vi "fpga_Sine Interpolation.vi"(6 "ready for output":bool, 8 "input valid":bool, 10 "Fnom":T1 items=["Fnom=50Hz", "Fnom=60Hz"], 11 "tach input":fxp<+/-,24,3> format="%.26g") -> (0 "output valid":bool, 1 "resampling valid":bool, 2 "crossing":fxp<+,32,16> format="%.21g", 3 "frequency":fxp<+,32,8> format="%.27g", 4 "ready for input":bool)   [LabVIEW 2011, in "NI_EP_Resample_FPGA.lvlib"]
uses:
  <vilib>/addons/Electrical Power/PQ/Resampling/NI_EP_Resample_FPGA.lvlib
  <vilib>/addons/Electrical Power/PQ/Resampling/FPGA/subVIs/fpga_Typedef Fnom.ctl
  <vilib>/rvi/FXPMathLib/basic elements/FxpIntAccumulator/subVIs/nifxpmath_IntAccumulator_SimConfig.ctl
  <vilib>/rvi/FXPMathLib/FxpSub/subVIs/nifxpmath_Sub_SimConfig.ctl
  <vilib>/fxp/LVFixedPointQuantizationPolicyTypeDef.ctl
  <vilib>/fxp/LVFixedPointOverflowPolicyTypeDef.ctl
  <vilib>/rvi/FXPMathLib/FxpDiv/subVIs/nifxpmath_Div_SimConfig.ctl
  <vilib>/rvi/FXPMathLib/FxpSinAndCos/subVIs/nifxpmath_SinAndCos_SimConfig.ctl
  <vilib>/rvi/FXPMathLib/FxpAtan2/subVIs/nifxpmath_Atan2_SimConfig.ctl
  <vilib>/rvi/FXPMathLib/basic elements/FxpIntAccumulator/simVIs/DllFxpIntAccumulator_sub.vi
  <vilib>/rvi/FXPMathLib/FxpSub/simVIs/DllFxpSubTemp_sub.vi
  <vilib>/rvi/FXPMathLib/FxpDiv/simVIs/DllFxpDivTemp_sub.vi
  <vilib>/rvi/FXPMathLib/FxpSinAndCos/simVIs/DllFxpSinAndCosTemp_sub.vi
  <vilib>/rvi/FXPMathLib/FxpAtan2/simVIs/DllFxpAtan2Temp_sub.vi
  <vilib>/rvi/FXPMathLib/basic elements/FxpIntAccumulator/XNode/nifxpmath_IntAccumulator.xnode
  <vilib>/rvi/FXPMathLib/FxpSub/XNode/nifxpmath_Sub.xnode
  <vilib>/rvi/FXPMathLib/FxpDiv/XNode/nifxpmath_Div.xnode
  <vilib>/rvi/FXPMathLib/FxpSinAndCos/XNode/nifxpmath_SinAndCos.xnode
  <vilib>/rvi/FXPMathLib/basic elements/FxpDiscreteDelay/XNode/nifxpmath_DiscreteDelay.xnode
  <vilib>/rvi/FXPMathLib/FxpMul/XNode/nifxpmath_Multiplier.xnode
  <vilib>/rvi/FXPMathLib/FxpAtan2/XNode/nifxpmath_Atan2.xnode
  <vilib>/rvi/FXPMathLib/FxpAdd/XNode/nifxpmath_Add.xnode
  <vilib>/rvi/FXPMathLib/sim/FxpSim.dll
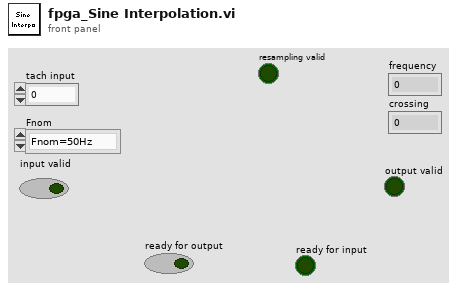
[diagram p1: front panel]
types:
  T1 = typedef "NI_EP_Resample_FPGA.lvlib/fpga_Typedef Fnom.ctl" = u8
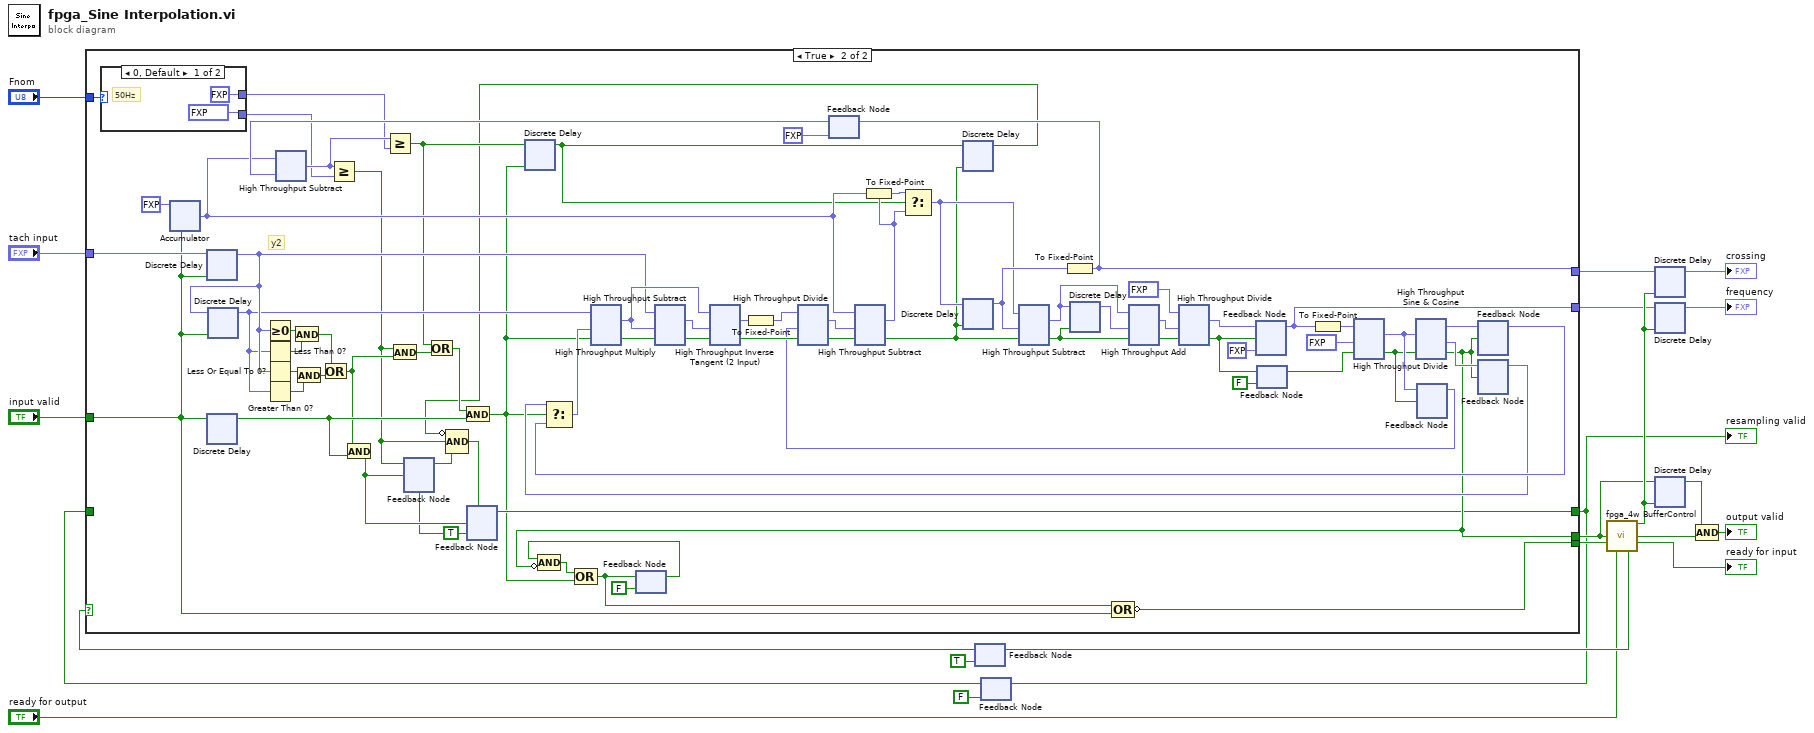
[diagram p0: block diagram]
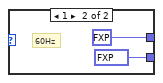
[diagram p3: hidden frame]
diagram:
  n1 = feedback #1(TRUE ("logic enable")) -> (w9:bool)
  n2 = feedback #2(FALSE ("logic enable")) -> (w4:bool)
  n3 = case shown="True" w9 {
    tunnel: "tach input" -> [_ w97]
    tunnel: "input valid" -> [_ w65]
    tunnel: [_ w52] -> w16
    tunnel: [_ w45] -> w14
    tunnel: [_ w39] -> w13
    tunnel: [_ w51] -> w12
    tunnel: "Fnom" -> [_ w38]
    tunnel: [w22 w33] -> w3
    tunnel: w4 -> [w22 _]
    frame False {
    }
    frame True {
      w23 = TRUE
      # "y2"
      n4 = case shown="0, Default" w38 {
        tunnel: [fxp<+,32,16> 25.0 ("y") fxp<+,32,16> 20.833328247070312 ("y")] -> w37
        tunnel: [fxp<+,32,16> 15.667007446289062 ("y") fxp<+,32,16> 12.889999389648438 ("y")] -> w36
        frame 0, Default {
          # "50Hz"
        }
        frame 1 {
          # "60Hz"
        }
      }
      n5 = xnode "Accumulator"("x"=fxp<+,16,16> 0.0, "carry-in/inverted borrow-in (F)"=w65) -> ("s"=w42:fxp<+,16,16>)  [unwired: 3 in, 1 out]
      n6 = xnode "Discrete Delay"("D"=w97, "enable"=w65) -> ("Q"=w67:fxp<+/-,24,3>)
      n7 = xnode "Discrete Delay"("D"=w65) -> ("Q"=w35:bool)
      n8 = xnode "Discrete Delay"("D"=w67, "enable"=w65) -> ("Q"=w66:fxp<+/-,24,3>)
      n9 = Greater Or Equal To 0?(x=w67) -> (x >= 0?=w73:bool)
      n10 = Less Than 0?(x=w66) -> (x < 0?=w72:bool)
      n11 = Less Or Equal To 0?(x=w67) -> (x <= 0?=w71:bool)
      n12 = Greater Than 0?(x=w66) -> (x > 0?=w70:bool)
      n13 = And(x=w73, y=w72) -> (x .and. y?=w69:bool)
      n14 = And(x=w71, y=w70) -> (x .and. y?=w68:bool)
      n15 = Or(x=w69, y=w68) -> (x .or. y?=w34:bool)
      n16 = And(x=w34, y=w35) -> (x .and. y?=w32:bool)
      n17 = feedback #3(w23) -> (w30:bool)
      n18 = feedback #4(w23) -> (w33:bool)
      n19 = feedback #5(FALSE) -> (w61:bool)
      n20 = feedback #6(fxp<+,32,16> 0.0) -> (w49:fxp<+,32,16>)
      n21 = xnode "High Throughput Subtract"("x"=w42, "y"=w49) -> ("x-y"=w48:fxp<+/-,32,16>)
      n22 = Greater Or Equal?(x=w48, y=w36) -> (x >= y?=w31:bool)
      n23 = Greater Or Equal?(x=w48, y=w37) -> (x >= y?=w27:bool)
      n24 = And(x=w31, y=w34) -> (x .and. y?=w47:bool)
      n25 = feedback-in #3(w31, w32) -> ()
      n26 = Or(x=w27, y=w47) -> (x .or. y?=w43:bool)
      n27 = And(x=w43, y=w35) -> (x .and. y?=w29:bool)
      n28 = xnode "Discrete Delay"("D"=w27, "enable"=w29) -> ("Q"=w25:bool)
      n29 = feedback #7(fxp<+,32,8> 50.0 ("x/y")) -> (w51:fxp<+,32,8>)
      n30 = feedback #8(FALSE ("output valid")) -> (w74:bool)
      n31 = To Fixed-Point(number=w51) -> (fixed-point=w75:fxp<+,16,8>)  [unwired: 1 in]
      n32 = xnode "High Throughput Divide"("x"=w75, "y"=fxp<+,7,10> 1000.0, "input valid"=w74) -> ("x/y"=w55:fxp<+,24,5>, "output valid"=w54:bool)  [unwired: 1 in, 1 out]
      n33 = xnode "High Throughput Sine & Cosine"("x (pi)"=w55, "input valid"=w54) -> ("sin(x)"=w59:fxp<+/-,24,2>, "cos(x)"=w58:fxp<+/-,24,2>, "output valid"=w45:bool)  [unwired: 1 in, 1 out]
      n34 = Compound Arithmetic op=AND(w61, invert w45) -> (w62:bool)
      n35 = Compound Arithmetic op=OR(w62, w29) -> (w60:bool)
      n36 = feedback-in #5(w60) -> ()
      n37 = Compound Arithmetic op=OR(w60, w65) -> (invert w52:bool)
      n38 = feedback #9() -> (w53:fxp<+,24,5>)  [unwired: 1 in]
      n39 = feedback-in #9(w55, w54) -> ()
      n40 = feedback #10() -> (w57:fxp<+/-,24,2>)  [unwired: 1 in]
      n41 = feedback-in #10(w59, w45) -> ()
      n42 = feedback #11() -> (w56:fxp<+/-,24,2>)  [unwired: 1 in]
      n43 = Select(t=w56, s=w29, f=w57) -> (s? t:f=w96:fxp<+/-,24,2>)
      n44 = xnode "High Throughput Multiply"("x"=w66, "y"=w96, "input valid"=w29) -> ("x*y"=w92:fxp<+/-,32,5>, "output valid"=w95:bool)  [unwired: 1 in, 1 out]
      n45 = xnode "High Throughput Subtract"("x"=w67, "y"=w92, "input valid"=w95) -> ("x-y"=w93:fxp<+/-,32,5>, "output valid"=w94:bool)  [unwired: 1 in, 1 out]
      n46 = xnode "High Throughput Inverse Tangent (2 Input)"("y"=w92, "x"=w93, "input valid"=w94) -> ("atan2(y,x) (pi)"=w89:fxp<+/-,32,2>, "output valid"=w88:bool)  [unwired: 1 in, 1 out]
      n47 = To Fixed-Point(number=w89) -> (fixed-point=w90:fxp<+/-,30,0>)  [unwired: 1 in]
      n48 = xnode "High Throughput Divide"("x"=w90, "y"=w53, "input valid"=w88) -> ("x/y"=w87:fxp<+/-,32,8>, "output valid"=w86:bool)  [unwired: 1 in, 1 out]
      n49 = xnode "High Throughput Subtract"("x"=w42, "y"=w87, "input valid"=w86) -> ("x-y"=w41:fxp<+,40,16>, "output valid"=w26:bool)  [unwired: 1 in, 1 out]
      n50 = To Fixed-Point(fixed-point type=w41, number=w42) -> (fixed-point=w40:fxp<+,40,16>)
      n51 = Select(t=w40, s=w25, f=w41) -> (s? t:f=w44:fxp<+,40,16>)
      n52 = xnode "Discrete Delay"("D"=w25, "enable"=w26) -> ("Q"=w24:bool)
      n53 = Compound Arithmetic op=AND(invert w24, w31, w30) -> (w28:bool)
      n54 = feedback-in #4(w28, w32) -> ()
      n55 = xnode "Discrete Delay"("D"=w44, "enable"=w26) -> ("Q"=w50:fxp<+,40,16>)
      n56 = xnode "High Throughput Subtract"("x"=w44, "y"=w50, "input valid"=w26) -> ("x-y"=w83:fxp<+,40,16>, "output valid"=w85:bool)  [unwired: 1 in, 1 out]
      n57 = To Fixed-Point(number=w50) -> (fixed-point=w39:fxp<+,32,16>)  [unwired: 1 in]
      n58 = feedback-in #6(w39) -> ()
      n59 = xnode "Discrete Delay"("D"=w83, "enable"=w85) -> ("Q"=w84:fxp<+,40,16>)
      n60 = xnode "High Throughput Add"("x"=w83, "y"=w84, "input valid"=w85) -> ("x+y"=w80:fxp<+,40,16>, "output valid"=w82:bool)  [unwired: 1 in, 1 out]
      n61 = xnode "High Throughput Divide"("x"=fxp<+,8,11> 2000.0 ("y"), "y"=w80, "input valid"=w82) -> ("x/y"=w79:fxp<+,32,8>, "output valid"=w78:bool)  [unwired: 1 in, 1 out]
      n62 = feedback-in #7(w79, w78) -> ()
      n63 = feedback-in #8(w78) -> ()
      n64 = feedback-in #11(w58, w45) -> ()
    }
  }
  "resampling valid" <- w3
  n65 = feedback-in #2(w3) -> ()
  n66 = call <vilib>:"fpga_4w BufferControl.vi"("DR"=w14, "RFI"=w16, "RFO"="ready for output") -> ("buff enable"=w17:bool, "output valid"=w18:bool, "ready for input"=→"ready for input":bool, "logic enable"=w10:bool)  [unwired: 9 in]
  n67 = feedback-in #1(w10) -> ()
  n68 = xnode "Discrete Delay"("D"=w13, "enable"=w17) -> ("Q"=→"crossing":fxp<+,32,16>)
  n69 = xnode "Discrete Delay"("D"=w12, "enable"=w17) -> ("Q"=→"frequency":fxp<+,32,8>)
  n70 = xnode "Discrete Delay"("D"=w14, "enable"=w17) -> ("Q"=w19:bool)
  n71 = Compound Arithmetic op=AND(w19, w18) -> (→"output valid":bool)
